vi "Shooter Motors.vi"(2 "Return":bool, 3 "Encoder":dbl, 4 "Fire":bool, 5 "State Control":enum16{"Open", "Run", "End"}(ring)) -> (0 "Fully retracted?":bool, 1 "Fully shot?":bool)   [LabVIEW 2013]
uses:
  <vilib>/Rock Robotics/SystemInterfaces/DIO/FPGA_DIOPWMChannel.ctl
  <vilib>/Rock Robotics/WPI/MotorControl/WPI_MotorControlOpen Talon.vi
panel:
  in  "rest":dbl=0.1 format="%#_13g"
  in  "Break point":dbl=20.0 format="%#_13g"
  in  "Break":dbl=-0.5 format="%#_13g"
  in  "Shoot":dbl=0.5 format="%#_13g"
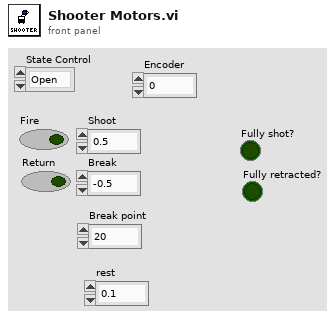
[diagram p1: front panel]
types:
  T1 = typedef "FPGA_DIOPWMChannel.ctl" = enum8{"PWM 1", "PWM 2", "PWM 3", "PWM 4", "PWM 5", "PWM 6", "PWM 7", "PWM 8", "PWM 9", "PWM 10", "Invalid"}
  T2 = typedef "WPI_MotorControlDeviceRef.ctl" = cluster{"DeviceStatus":errorcluster, "Type":enum16{"PWM", "CAN"}, "PWM":cluster{"Digital Module":T3, "PWM Channel":T1, "DeadBand":T4}, "CAN":cluster{"Device Number":u8, "Control Mode":T5, "Semaphore":T6, "Max Vout":dbl}, "Invert":bool, "TransformRef":T7, "InvTransformRef":T7}
  T3 = typedef "FPGA_TypedefDigitalModule.ctl" = enum16{"Digital Module 1", "Digital Module 2"}
  T4 = typedef "WPI_PWMDeadband.ctl" = cluster{"Name":string, "maxPositivePwm":i32, "minPositivePwm":i32, "centerPwm":i32, "maxNegativePwm":i32, "minNegativePwm":i32, "angularRange":u16}
  T5 = typedef "WPI_CANJaguar_ControlMode.ctl" = enum8{"Percent VBus", "Current", "Speed", "Position", "Voltage"}
  T6 = typedef "Semaphore RefNum" = refnum<k1>
  T7 = typedef "WPI_PWMTransform_ConPane.ctl" = refnum<vi>
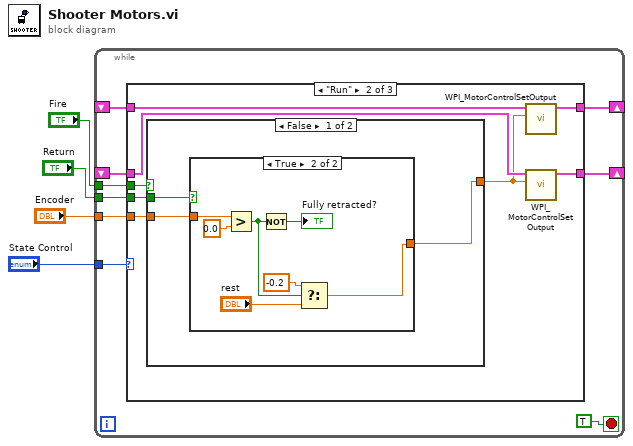
[diagram p0: block diagram]
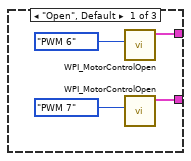
[diagram p2: hidden frame]
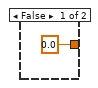
[diagram p3: hidden frame]
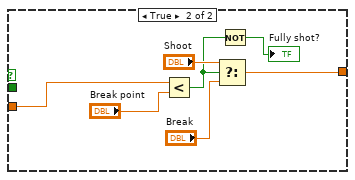
[diagram p4: hidden frame]
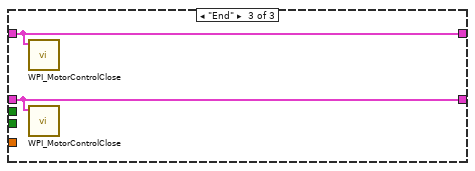
[diagram p5: hidden frame]
diagram:
  n1 = while {
    shift-right: [w13] -> _
    shift-left: _ -> [w12]
    tunnel: "State Control" -> [w11]
    shift-right: [w9] -> _
    shift-left: _ -> [w8]
    tunnel: "Fire" -> [w7]
    tunnel: "Return" -> [w6]
    tunnel: "Encoder" -> [w5]
    stop <- TRUE stop-if-true
    n2 = case shown="\"Run\"" w11 {
      tunnel: [w15 w22 w45] -> w13
      tunnel: w12 -> [_ w24 w45]
      tunnel: [w14 w21 w44] -> w9
      tunnel: w8 -> [_ w25 w44]
      tunnel: w7 -> [_ w20 _]
      tunnel: w6 -> [_ w19 _]
      tunnel: w5 -> [_ w18 _]
      frame "Open", Default {
        n3 = call-poly <vilib>:"WPI_MotorControlOpen.vi"("PWM Channel"=FPGA_DIOPWMChannel."PWM 6" ("PWMChannel")) -> ("MotorControlDeviceRef"=w15:T2)  [unwired: 9 in, 1 out]
        n4 = call-poly <vilib>:"WPI_MotorControlOpen.vi"("PWM Channel"=FPGA_DIOPWMChannel."PWM 7" ("PWMChannel")) -> ("MotorControlDeviceRef"=w14:T2)  [unwired: 9 in, 1 out]
      }
      frame "Run" {
        n5 = case shown="False" w20 {
          tunnel: [w27 w40] -> w23
          tunnel: w19 -> [w28 _]
          tunnel: w18 -> [w26 w39]
          frame False {
            n6 = case shown="True" w28 {
              tunnel: [0.0 w32] -> w27
              tunnel: w26 -> [_ w36]
              frame False {
              }
              frame True {
                n7 = Greater?(x=w36, y=0.0) -> (0:w31:bool)
                n8 = Not(x=w31) -> (.not. x?=→"Fully retracted?":bool)
                n9 = Select(t=-0.2, s=w31, f="rest") -> (s? t:f=w32:dbl)
              }
            }
          }
          frame True {
            n10 = Less?(x=w39, y="Break point") -> (x < y?=w38:bool)
            n11 = Select(t="Shoot", s=w38, f="Break") -> (s? t:f=w40:dbl)
            n12 = Not(x=w38) -> (.not. x?=→"Fully shot?":bool)
          }
        }
        n13 = call <vilib>:"WPI_MotorControlSetOutput.vi"("Output"=w23, "MotorControlDevRef"=w24) -> ("MotorControlDevRef"=w22:T2)  [unwired: 7 in, 2 out]
        n14 = call <vilib>:"WPI_MotorControlSetOutput.vi"("Output"=w23, "MotorControlDevRef"=w25) -> ("MotorControlDevRef"=w21:T2)  [unwired: 7 in, 2 out]
      }
      frame "End" {
        n15 = call <vilib>:"WPI_MotorControlClose.vi"("MotorControlDevRef"=w45) -> ()  [unwired: 10 in, 1 out]
        n16 = call <vilib>:"WPI_MotorControlClose.vi"("MotorControlDevRef"=w44) -> ()  [unwired: 10 in, 1 out]
      }
    }
  }
